vi "MotorWatch.vi"(11 "Setpoint":dbl) -> ()   [LabVIEW 2016]
uses:
  Robot Global Data.vi
panel:
  out "Waveform Chart 2":dbl(graph)
  out "Avg Val":dbl
  out "Waveform Chart":dbl(graph)
  out "Degrees per Second":dbl
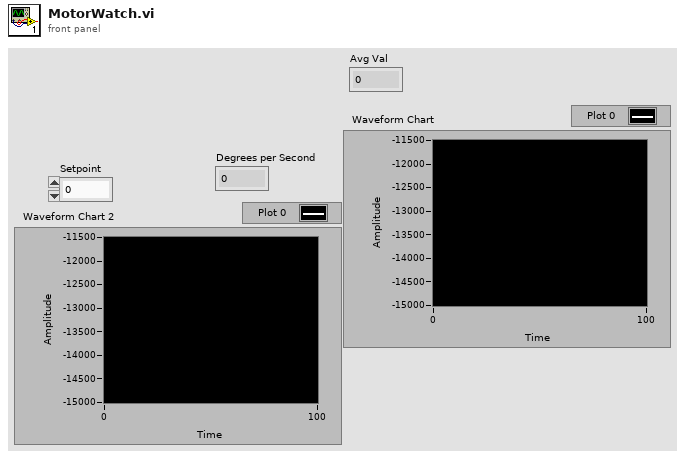
[diagram p1: front panel]
types:
  T1 = typedef "WPI_EncoderDevRef.ctl" = cluster{"DevStatus":errorcluster, "EncoderIndex":T2, "CounterIndex":T3, "DistancePerCount":dbl, "Decoding Type":T4}
  T2 = typedef "FPGA_EncoderIdx.ctl" = enum8{"Enc 0", "Enc 1", "Enc 2", "Enc 3", "Enc 4", "Enc 5", "Enc 6", "Enc 7", "Invalid"}
  T3 = typedef "FPGA_CounterCtrSystemIndex.ctl" = enum8{"Ctr 0", "Ctr 1", "Ctr 2", "Ctr 3", "Ctr 4", "Ctr 5", "Ctr 6", "Ctr 7", "Invalid"}
  T4 = typedef "WPI_EncoderType.ctl" = enum16{"1x", "2x", "4x"}
  T5 = typedef "WPI_MotorControlDeviceRef.ctl" = cluster{"DeviceStatus":errorcluster, "Type":T6, "PWM":cluster{"PWM Channel":T7, "DeadBand":T8}, "CAN":cluster{"Device Number":u8, "SetOutput VI Ref":variant, "GetOutput VI Ref":variant, "Enable VI Ref":variant, "Disable VI Ref":variant, "Data":variant}, "Invert":bool}
  T6 = typedef "WPI_MotorControlType.ctl" = enum16{"PWM", "CAN"}
  T7 = typedef "FPGA_DIOPWMChannel.ctl" = enum8{"PWM 0", "PWM 1", "PWM 2", "PWM 3", "PWM 4", "PWM 5", "PWM 6", "PWM 7", "PWM 8", "PWM 9", "PWM MXP 0", "PWM MXP 1", "PWM MXP 2", "PWM MXP 3", "PWM MXP 4", "PWM MXP 5", "PWM MXP 6", "PWM MXP 7", "PWM MXP 8", "PWM MXP 9", "Invalid"}
  T8 = typedef "WPI_PWMDeadband.ctl" = cluster{"Name":string, "maxPositivePwm":i32, "minPositivePwm":i32, "centerPwm":i32, "maxNegativePwm":i32, "minNegativePwm":i32, "angularRange":u16}
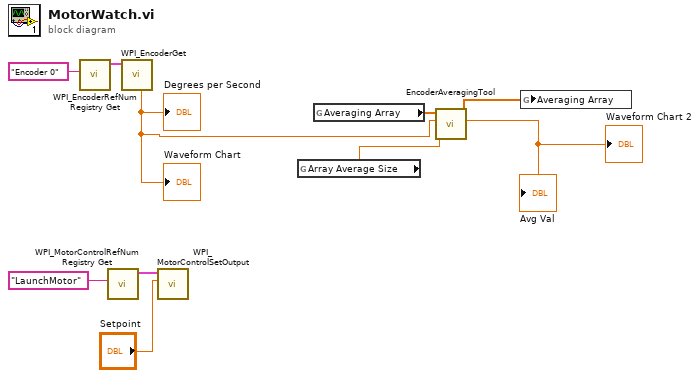
[diagram p0: block diagram]
diagram:
  n1 = call <vilib>:"WPI_EncoderRefNum Registry Get.vi"("refnum name"="Encoder 0") -> ("EncoderDevRef"=w6:T1)  [unwired: 9 in, 1 out]
  n2 = call <vilib>:"WPI_MotorControlRefNum Registry Get.vi"("refnum name"="LaunchMotor") -> ("MotorControlDevRef"=w9:T5)  [unwired: 9 in, 1 out]
  n3 = call <vilib>:"WPI_EncoderGet.vi"("EncoderDevRef"=w6) -> ("Rate"=w3:dbl)  [unwired: 5 in, 5 out]
  "Degrees per Second" <- w3
  "Waveform Chart" <- w3
  n4 = call <vilib>:"WPI_MotorControlSetOutput.vi"("Output"="Setpoint", "MotorControlDevRef"=w9) -> ()  [unwired: 7 in, 3 out]
  n5 = global read "Robot Global Data.vi" "Array Average Size"() -> (w2:dbl)
  n6 = global read "Robot Global Data.vi" "Averaging Array"() -> (w5:dbl[])
  n7 = call "EncoderAveragingTool.vi"("Avg Size"=w2, "Reading"=w3, "Array"=w5) -> ("Avg Val"=→"Avg Val" →"Waveform Chart 2":dbl, "Array 2"=w4:dbl[])  [unwired: 7 in]
  n8 = global write "Robot Global Data.vi" "Averaging Array"(w4) -> ()
